vi "Init - Setup Duplex.vi"(8 "error in (no error)":errorcluster, 11 "Compiled.Settings in":T1 {"Tx Packet Info"."targetPriority" min=1 step=1; "Tx Packet Info"."targetProcessor" min=-2 max=16 step=1; "Tx Packet Info"."Endianness" items=["big-endian"=0, "little-indian"=2]; "Rx Packet Info"."Endianness" items=["big-endian"=0, "little-indian"=2]}) -> (0 "error out":errorcluster, 3 "Compiled.Settings out":T1 {"Tx Packet Info"."targetPriority" min=1 step=1; "Tx Packet Info"."targetProcessor" min=-2 max=16 step=1; "Tx Packet Info"."Endianness" items=["big-endian"=0, "little-indian"=2]; "Rx Packet Info"."Endianness" items=["big-endian"=0, "little-indian"=2]})   [LabVIEW 2016, in "UDP-Custom-Device Engine.lvlib"]
uses:
  UDP-Custom-Device Engine.lvlib
  Shared/Compiled.Settings.ctl
  Shared/Types/Shared - Rx.PacketInfo.ctl
  Shared/Types/Shared - Channel Data Type.ctl
  Shared/Types/Shared - Buffered.PacketInfo.ctl
  Shared/Types/Shared - Pointer Encoding.ctl
  Shared/Types/Shared - Receive Buffer Options.ctl
  Shared/Types/Shared - Transmit Buffer Options.ctl
  Shared/Types/Shared - Duplex Settings.ctl
  Shared/Types/Shared - New Data Options.ctl
  Shared/Types/Shared - Tx.PacketInfo.ctl
  Shared/Types/Shared - Transmit Flag Options.ctl
  Shared/Types/Shared - Transmit Echo Options.ctl
  Shared/Types/Shared - Transmit Sim Options.ctl
  Shared/Types/Shared - Header Details.ctl
  <vilib>/Utility/tcp.llb/UDP Multicast Read-Write Open.vi
  Shared/UDP-Custom-Device Shared.lvlib
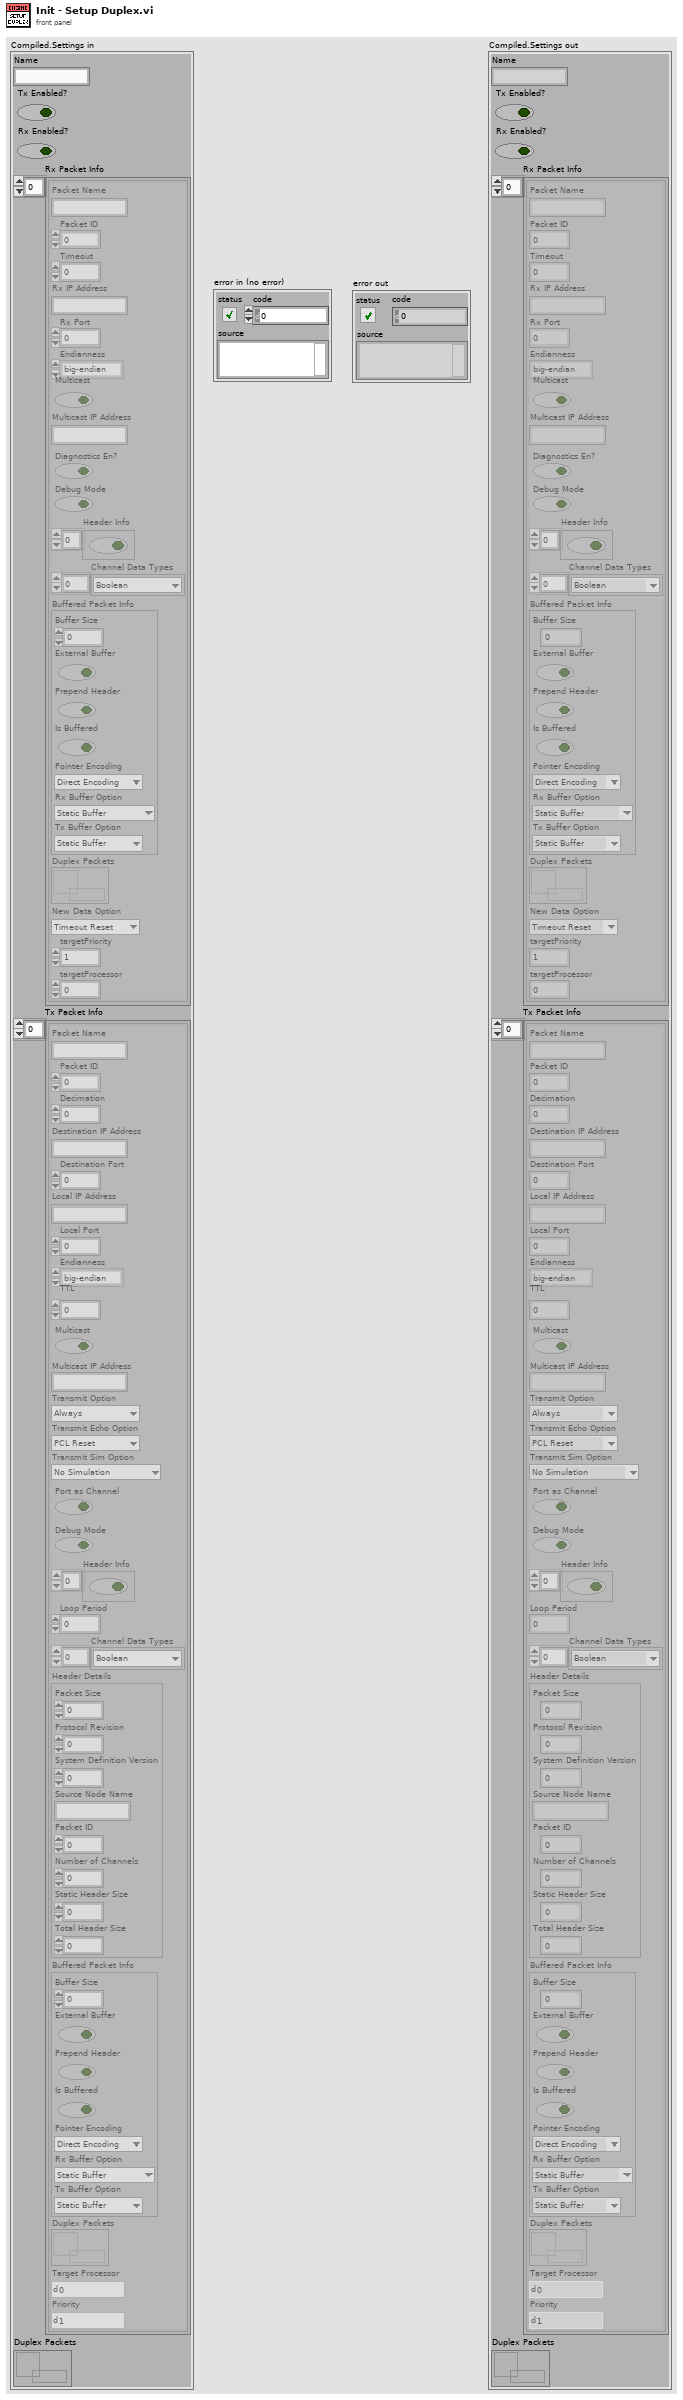
[diagram p1: front panel]
types:
  T1 = typedef "UDP-Custom-Device Shared.lvlib/Compiled.Settings.ctl" = cluster{"Name":string, "Tx Enabled?":bool, "Rx Enabled?":bool, "Rx Packet Info":T2[], "Tx Packet Info":T9[], "Duplex Packets":refnum<data-value>}
  T2 = typedef "UDP-Custom-Device Shared.lvlib/Shared - Rx.PacketInfo.ctl" = cluster{"Packet Name":string, "Packet ID":i32, "Timeout":i32, "Rx IP Address":string, "Rx Port":u16, "Endianness":u16, "Multicast":bool, "Multicast IP Address":string, "Diagnostics En?":bool, "Debug Mode":bool, "Header Info":bool[], "Channel Data Types":T3[], "Buffered Packet Info":T4, "Duplex Packets":refnum<data-value>, "New Data Option":T8, "targetPriority":i16, "targetProcessor":i8}
  T3 = typedef "UDP-Custom-Device Shared.lvlib/Shared - Channel Data Type.ctl" = enum16{"Boolean", "Single", "Double", "I8", "I16", "I32", "I64", "U8", "U16", "U32", "U64"}
  T4 = typedef "UDP-Custom-Device Shared.lvlib/Shared - Buffered.PacketInfo.ctl" = cluster{"Buffer Size":i32, "External Buffer":bool, "Prepend Header":bool, "Is Buffered":bool, "Pointer Encoding":T5, "Rx Buffer Option":T6, "Tx Buffer Option":T7}
  T5 = typedef "UDP-Custom-Device Shared.lvlib/Shared - Pointer Encoding.ctl" = enum16{"Direct Encoding", "Conversion Encoding"}
  T6 = typedef "UDP-Custom-Device Shared.lvlib/Shared - Receive Buffer Options.ctl" = enum16{"Static Buffer", "Circular Buffer", "Circular Buffer + Size"}
  T7 = typedef "UDP-Custom-Device Shared.lvlib/Shared - Transmit Buffer Options.ctl" = enum16{"Static Buffer", "FIFO Buffer", "FIFO Buffer + Port"}
  T8 = typedef "UDP-Custom-Device Shared.lvlib/Shared - New Data Options.ctl" = enum16{"Timeout Reset", "Counter"}
  T9 = typedef "UDP-Custom-Device Shared.lvlib/Shared - Tx.PacketInfo.ctl" = cluster{"Packet Name":string, "Packet ID":i32, "Decimation":u16, "Destination IP Address":string, "Destination Port":u16, "Local IP Address":string, "Local Port":u16, "Endianness":u16, "TTL":u16, "Multicast":bool, "Multicast IP Address":string, "Transmit Option":T10, "Transmit Echo Option":T11, "Transmit Sim Option":T12, "Port as Channel":bool, "Debug Mode":bool, "Header Info":bool[], "Loop Period":u32, "Channel Data Types":T3[], "Header Details":T13, "Buffered Packet Info":T4, "Duplex Packets":refnum<data-value>, "targetProcessor":i8, "targetPriority":i16}
  T10 = typedef "UDP-Custom-Device Shared.lvlib/Shared - Transmit Flag Options.ctl" = enum16{"Always", "One-Shot", "Toggle"}
  T11 = typedef "UDP-Custom-Device Shared.lvlib/Shared - Transmit Echo Options.ctl" = enum16{"PCL Reset", "Counter", "Mirror"}
  T12 = typedef "UDP-Custom-Device Shared.lvlib/Shared - Transmit Sim Options.ctl" = enum16{"No Simulation", "Counter", "Full Buffer", "FIFO Test", "FIFO + Port Test"}
  T13 = typedef "UDP-Custom-Device Shared.lvlib/Shared - Header Details.ctl" = cluster{"Packet Size":u16, "Protocol Revision":u8, "System Definition Version":u64, "Source Node Name":string, "Packet ID":u32, "Number of Channels":u32, "Static Header Size":u16, "Total Header Size":u16}
  T14 = typedef "UDP-Custom-Device Shared.lvlib/Shared - Duplex Settings.ctl" = cluster{"Transmit Packet ID":i32, "Receive Packet ID":i32, "Multicast":bool, "Multicast Address":string, "IP Address":string, "Port":u16, "TTL":u16, "Duplex Connection":refnum<k16>}
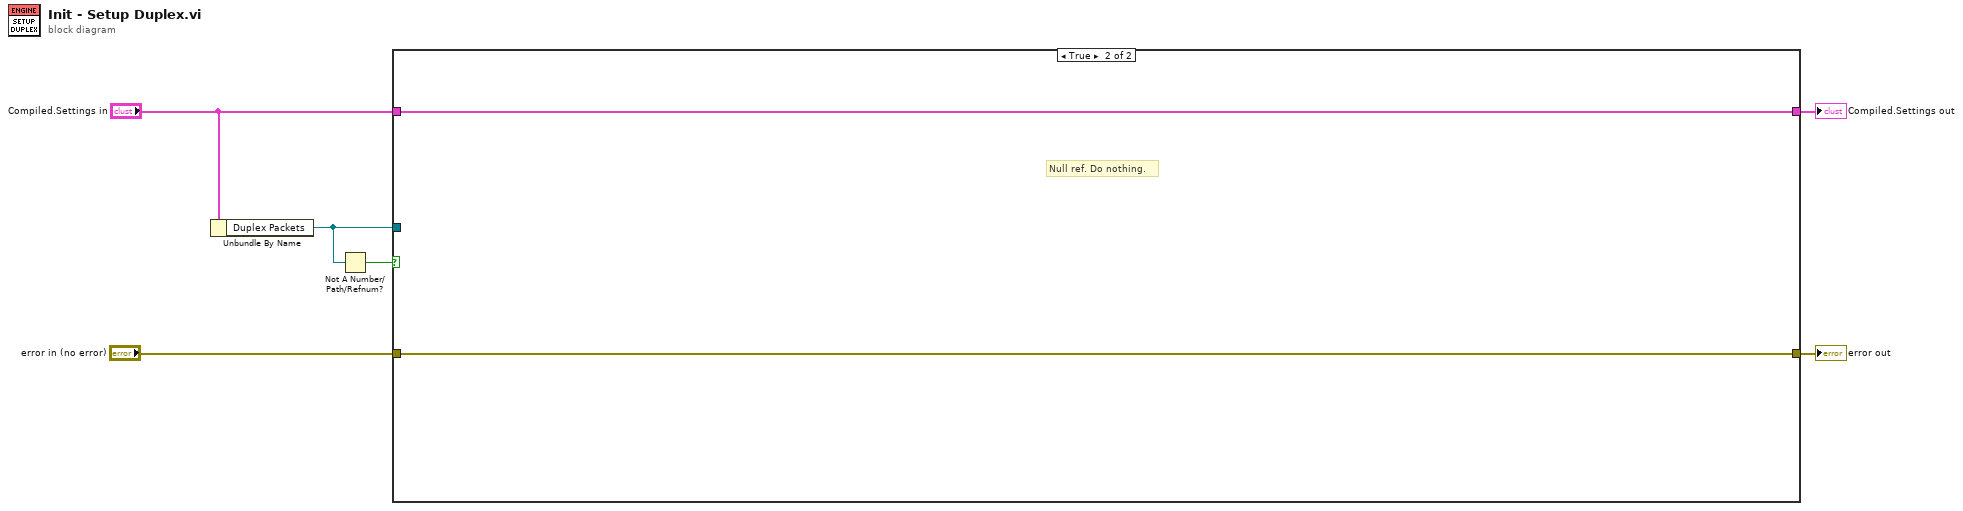
[diagram p0: block diagram]
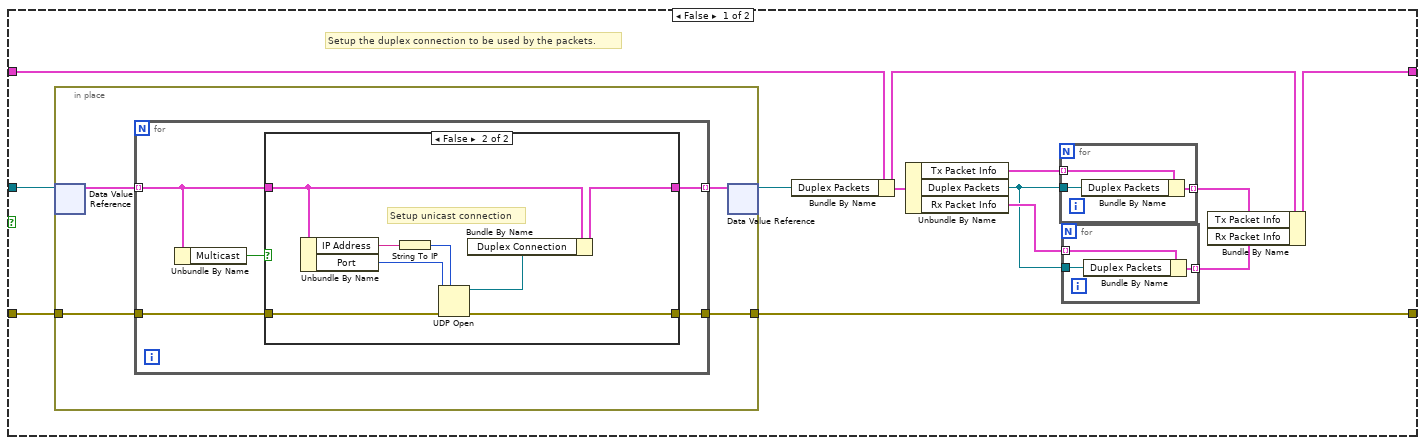
[diagram p2: hidden frame]
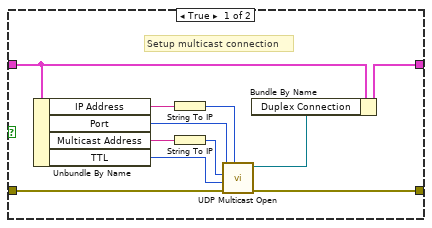
[diagram p3: hidden frame]
diagram:
  n1 = Unbundle By Name("Compiled.Settings in") -> ("Duplex Packets"=w2:refnum<data-value>)
  n2 = Not A Number/Path/Refnum?(number/path/refnum=w2) -> (NaN/Path/Refnum?=w1:bool)
  n3 = case shown="True" w1 {
    tunnel: "Compiled.Settings in" -> [w18 w54]
    tunnel: "error in (no error)" -> [w17 w53]
    tunnel: [w16 w53] -> w4
    tunnel: [w11 w54] -> w3
    tunnel: w2 -> [w14 _]
    frame False {
      # "Setup the duplex connection to be used by the packets."
      n4 = in-place {
        in-place-border: w17 -> [w28]
        in-place-border: [w27] -> w16
        n5 = in-place-dvr #1(w14) -> (w26:T14[])  [unwired: 1 out]
        n6 = for {
          tunnel: w26 -> [w32] mode=indexing
          tunnel: w28 -> [w31]
          tunnel: [w30] -> w25 mode=indexing
          tunnel: [w29] -> w27
          n7 = Unbundle By Name(w32) -> ("Multicast"=w33:bool)
          n8 = case shown="False" w33 {
            tunnel: w32 -> [w37 w48]
            tunnel: w31 -> [w44 w52]
            tunnel: [w36 w47] -> w30
            tunnel: [w34 w45] -> w29
            frame True {
              # "Setup multicast connection"
              n9 = Unbundle By Name(w37) -> ("IP Address"=w42:string, "Port"=w38:u16, "Multicast Address"=w43:string, "TTL"=w39:u16)
              n10 = String To IP(1:w42) -> (0:w41:u32)
              n11 = String To IP(1:w43) -> (0:w40:u32)
              n12 = call-poly <vilib>:"UDP Multicast Open.vi"("net address"=w41, "error in (no error)"=w44, "time-to-live (1)"=w39, "multicast addr"=w40, "port"=w38) -> ("error out"=w34:errorcluster, "connection ID"=w35:refnum<k16>)  [unwired: 4 in, 1 out]
              n13 = Bundle By Name(cluster=w37, "Duplex Connection"=w35) -> (w36:T14)
            }
            frame False {
              # "Setup unicast connection"
              n14 = Unbundle By Name(w48) -> ("IP Address"=w51:string, "Port"=w49:u16)
              n15 = String To IP(1:w51) -> (0:w50:u32)
              n16 = UDP Open(7:w50, 8:w52, 11:w49) -> (port=w46:refnum<k16>, 0:w45:errorcluster)  [unwired: 2 in, 1 out]
              n17 = Bundle By Name(cluster=w48, "Duplex Connection"=w46) -> (w47:T14)
            }
          }
        }
        n18 = in-place-dvr #1(w25) -> (w15:refnum<data-value>)  [unwired: 1 out]
      }
      n19 = Bundle By Name(cluster=w18, "Duplex Packets"=w15) -> (w12:T1)
      n20 = Unbundle By Name(w12) -> ("Tx Packet Info"=w13:T9[], "Duplex Packets"=w8:refnum<data-value>, "Rx Packet Info"=w9:T2[])
      n21 = for {
        tunnel: w13 -> [w24] mode=indexing
        tunnel: w8 -> [w23]
        tunnel: [w22] -> w10 mode=indexing
        n22 = Bundle By Name(cluster=w24, "Duplex Packets"=w23) -> (w22:T9)
      }
      n23 = for {
        tunnel: w9 -> [w21] mode=indexing
        tunnel: w8 -> [w20]
        tunnel: [w19] -> w7 mode=indexing
        n24 = Bundle By Name(cluster=w21, "Duplex Packets"=w20) -> (w19:T2)
      }
      n25 = Bundle By Name(cluster=w12, "Tx Packet Info"=w10, "Rx Packet Info"=w7) -> (w11:T1)
    }
    frame True {
      # "Null ref. Do nothing."
    }
  }
  "Compiled.Settings out" <- w3
  "error out" <- w4
